vi "stop_tasks.vi"(0 "Counter (in)":refnum<class "Counter.lvclass">, 1 "Analog_Output (in)":refnum<class "Analog_Output.lvclass">, 3 "HSDIO (in)":refnum<class "HSDIO.lvclass">, 4 "DAQmx_pulse_out (in)":refnum<class "DAQmx_pulse_out.lvclass">, 5 "error in":errorcluster) -> (14 "Counter":refnum<class "Counter.lvclass">, 15 "Analog_Output":refnum<class "Analog_Output.lvclass">, 17 "HSDIO":refnum<class "HSDIO.lvclass">, 18 "DAQmx_pulse":refnum<class "DAQmx_pulse_out.lvclass">, 19 "error out":errorcluster)   [LabVIEW 2013]
uses:
  HSDIO/HSDIO.lvclass
  DAQmx_pulse_out/DAQmx_pulse_out.lvclass
  Analog_output/Analog_Output.lvclass
  Counter/Counter.lvclass
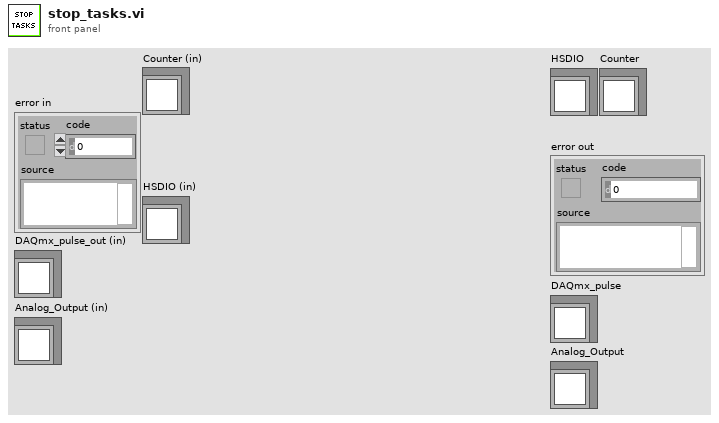
[diagram p1: front panel]
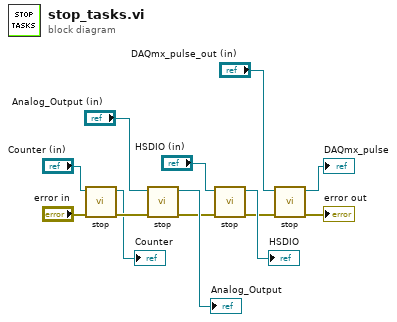
[diagram p0: block diagram]
diagram:
  n1 = call-dynamic "stop.vi"("error in (no error)"="error in", "Counter in"="Counter (in)") -> ("error out"=w3:errorcluster, "Counter out"=→"Counter":refnum<class "Counter.lvclass">)  [unwired: 8 in]
  n2 = call-dynamic "stop.vi"("error in (no error)"=w3, "Analog_Output in"="Analog_Output (in)") -> ("error out"=w5:errorcluster, "Analog_Output out"=→"Analog_Output":refnum<class "Analog_Output.lvclass">)  [unwired: 8 in]
  n3 = call-dynamic "stop.vi"("error in (no error)"=w5, "HSDIO in"="HSDIO (in)") -> ("error out"=w11:errorcluster, "HSDIO out"=→"HSDIO":refnum<class "HSDIO.lvclass">)  [unwired: 8 in]
  n4 = call-dynamic "stop.vi"("error in (no error)"=w11, "DAQmx_pulse_out in"="DAQmx_pulse_out (in)") -> ("error out"=→"error out":errorcluster, "DAQmx_pulse_out out"=→"DAQmx_pulse":refnum<class "DAQmx_pulse_out.lvclass">)  [unwired: 8 in]
